vi "Queued State Machine.vi"   [LabVIEW 2020, in "State Machine.lvlib"]
uses:
  State Machine.lvlib
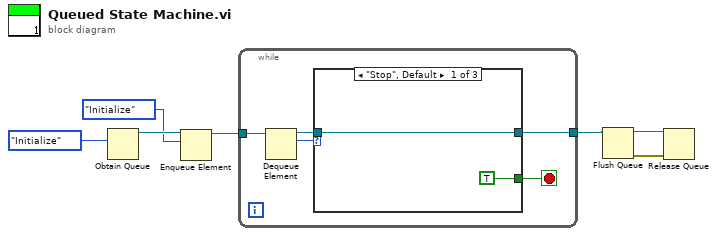
[diagram p0: block diagram]
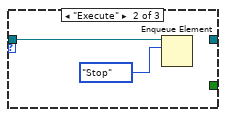
[diagram p2: hidden frame]
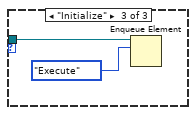
[diagram p3: hidden frame]
diagram:
  n1 = Obtain Queue(element data type=enum16{"Stop", "Execute", "Initialize"}."Initialize") -> (queue out=w6:refnum<queue>)  [unwired: 4 in, 2 out]
  n2 = Enqueue Element(queue=w6, element=enum16{"Stop", "Execute", "Initialize"}."Initialize") -> (queue out=w4:refnum<queue>)  [unwired: 2 in, 2 out]
  n3 = while {
    tunnel: w4 -> [w12]
    tunnel: [w8] -> w3
    stop <- w9 stop-if-true
    n4 = Dequeue Element(queue=w12) -> (queue out=w10:refnum<queue>, element=w11:enum16{"Stop", "Execute", "Initialize"})  [unwired: 2 in, 2 out]
    n5 = case shown="\"Stop\", Default" w11 {
      tunnel: w10 -> [w13 w16 w17]
      tunnel: [TRUE _ _] -> w9
      tunnel: [w13 _ _] -> w8
      frame "Stop", Default {
      }
      frame "Execute" {
        n6 = Enqueue Element(queue=w16, element=enum16{"Stop", "Execute", "Initialize"}."Stop") -> ()  [unwired: 2 in, 3 out]
      }
      frame "Initialize" {
        n7 = Enqueue Element(queue=w17, element=enum16{"Stop", "Execute", "Initialize"}."Execute") -> ()  [unwired: 2 in, 3 out]
      }
    }
  }
  n8 = Flush Queue(queue=w3) -> (queue out=w2:refnum<queue>, error out=w1:errorcluster)  [unwired: 1 in, 1 out]
  n9 = Release Queue(queue=w2, error in (no error)=w1) -> ()  [unwired: 1 in, 3 out]
